vi "Configure Measurement (Spurious Emissions).vi"(0 "VISA resource name":refnum<visa-resource-name>, 5 "Spurious Report Mode (0: All)":i32(ring) items=["All", "Limit"], 7 "Measurement Type (0: Examine)":i32(ring) items=["Examine", "Full"], 9 "Spur Number (1)":i32=1 format="%.0g", 11 "error in (no error)":errorcluster) -> (4 "VISA resource name out":refnum<visa-resource-name>, 15 "error out":errorcluster)   [LabVIEW 2018, in "Agilent MXA Series.lvlib"]
doc: "Sets the Spurious Emissions measurement parameters."
uses:
  Agilent MXA Series.lvlib
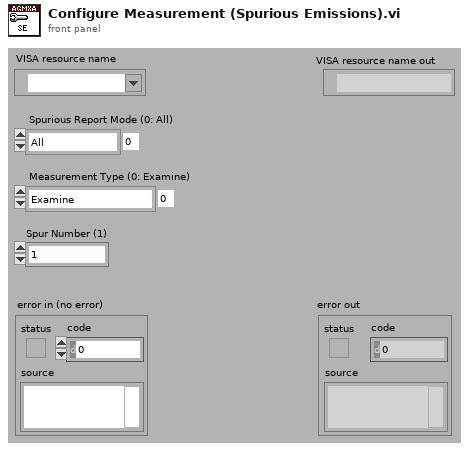
[diagram p1: front panel]
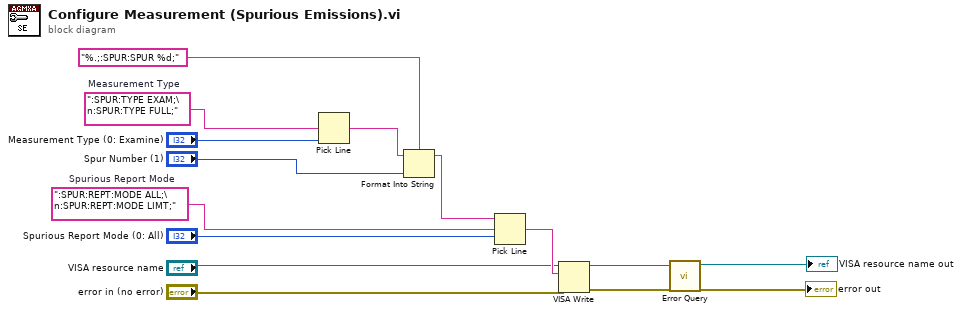
[diagram p0: block diagram]
diagram:
  w7 = ":SPUR:REPT:MODE ALL;\n:SPUR:REPT:MODE LIMT;"  # Spurious Report Mode
  w12 = ":SPUR:TYPE EXAM;\n:SPUR:TYPE FULL;"  # Measurement Type
  n1 = Pick Line(multi-line string=w12, line index="Measurement Type (0: Examine)") -> (output string=w11:string)  [unwired: 1 in]
  n2 = Format Into String(format string="%.;:SPUR:SPUR %d;", initial string=w11, "Spur Number (1)") -> (resulting string=w6:string)  [unwired: 1 in, 1 out]
  n3 = Pick Line(string ("")=w6, multi-line string=w7, line index="Spurious Report Mode (0: All)") -> (output string=w5:string)
  n4 = VISA Write(VISA resource name="VISA resource name", write buffer=w5, error in (no error)="error in (no error)") -> (VISA resource name out=w14:refnum<visa-resource-name>, error out=w15:errorcluster)  [unwired: 1 out]
  n5 = call "Error Query.vi"("error in (no error)"=w15, "VISA resource name"=w14) -> ("error out"=→"error out":errorcluster, "VISA resource name out"=→"VISA resource name out":refnum<visa-resource-name>)  [unwired: 6 in, 2 out]
